vi "FXP Raw to DBL.vi"(7 "FXP Configuration":T1, 8 "error in (no error)":errorcluster, 10 "Bool Data":bool[](array[boolean])) -> (0 "error out":errorcluster, 2 "DBL Value":dbl)   [LabVIEW 2026, in "FPGA Register IO.lvlib"]
uses:
  FPGA Register IO.lvlib
  TypeDefs/FXP Configuration.ctl
  <vilib>/fxp/LVFixedPointRepBitsTypeDef.ctl
  <vilib>/fxp/LVFixedPointRepRangeTypeDef.ctl
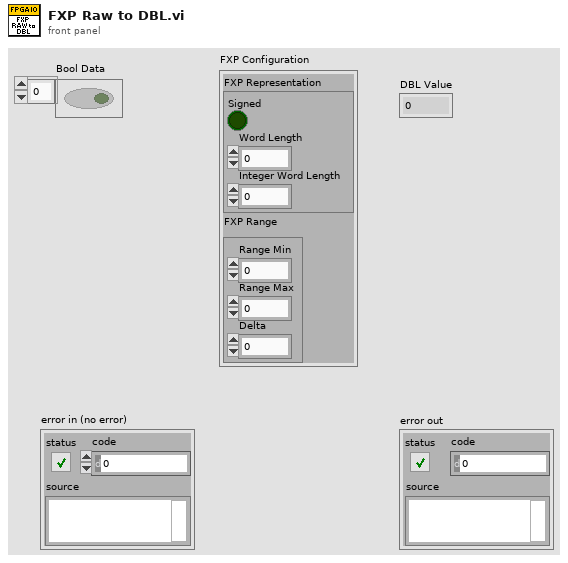
[diagram p1: front panel]
types:
  T1 = typedef "FPGA Register IO.lvlib/FXP Configuration.ctl" = cluster{"FXP Representation":T2, "FXP Range":T3}
  T2 = typedef "LVFixedPointRepBitsTypeDef.ctl" = cluster{"Signed":bool, "Word Length":u32, "Integer Word Length":i32}
  T3 = typedef "LVFixedPointRepRangeTypeDef.ctl" = cluster{"Range Min":dbl, "Range Max":dbl, "Delta":dbl}
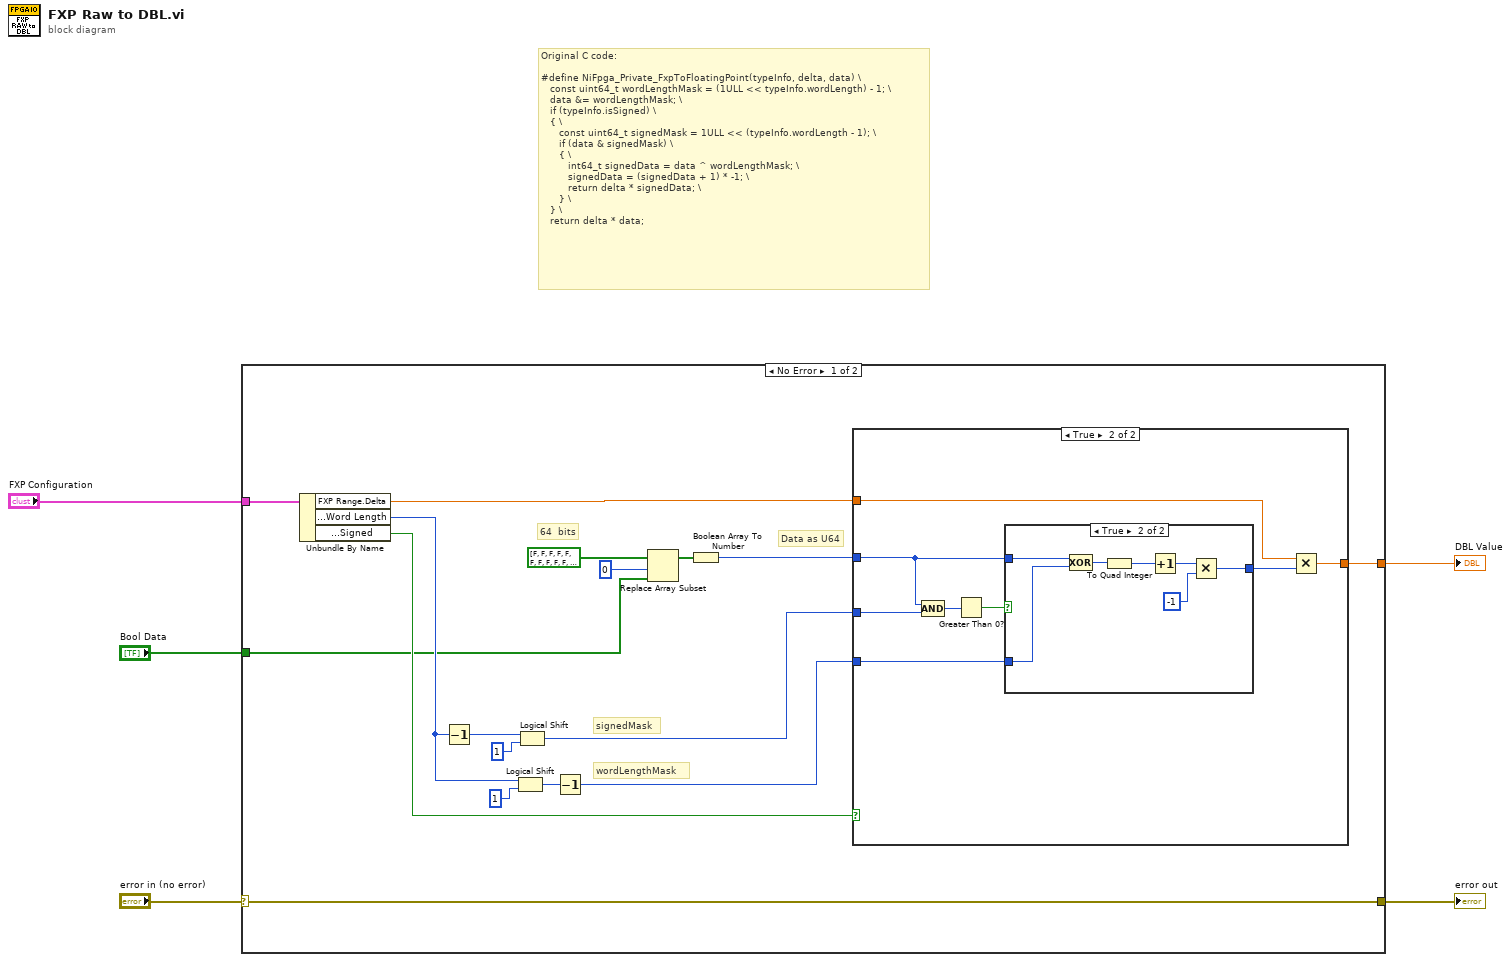
[diagram p0: block diagram]
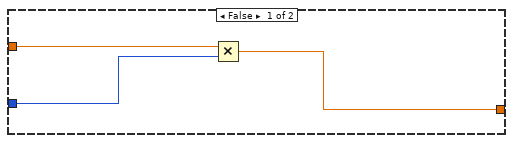
[diagram p2: hidden frame]
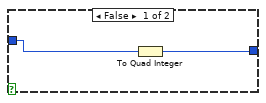
[diagram p3: hidden frame]
diagram:
  # "Original C code: \n\n#define NiFpga_Private_FxpToFloatingPoint(typeInfo, delta, data) \\\n   const uint64_t wordLengthMask = (1ULL << typeInfo.wordLength) - 1; \\\n   data &= wordLengthMask; \\\n   if (typeInfo.isSigned) \\\n   { \\\n      const uint64_t signedMask = 1ULL << (typeInfo.wordLength - 1); \\\n      if (data & signedMask) \\\n      { \\\n         int64_t signedData = data ^ wordLengthMask; \\\n         signedData = (signedData + 1) * -1; \\\n         return delta * signedData; \\\n      } \\\n   } \\\n   return delta * data;"
  n1 = case shown="No Error" "error in (no error)" {
    selector: "error in (no error)" -> [w10 w43]
    tunnel: "Bool Data" -> [w8 _]
    tunnel: [w15 _] -> w3
    tunnel: "FXP Configuration" -> [w14 _]
    tunnel: [w10 w43] -> w2
    frame No Error {
      # "wordLengthMask"
      # "signedMask"
      # "Data as U64"
      # "64  bits"
      n2 = Unbundle By Name(w14) -> ("FXP Range.Delta"=w13:dbl, "FXP Representation.Word Length"=w12:u32, "FXP Representation.Signed"=w11:bool)
      n3 = Decrement(x=w12) -> (x-1=w20:u32)
      n4 = Logical Shift(y=w12, x=u64 1) -> (x << y=w17:u64)
      n5 = Logical Shift(y=w20, x=u64 1) -> (x << y=w19:u64)
      n6 = Decrement(x=w17) -> (x-1=w16:u64)
      n7 = Replace Array Subset(array=bool[] [FALSE, FALSE, FALSE, FALSE, FALSE, FALSE, FALSE, FALSE, FALSE, FALSE, FALSE, FALSE, FALSE, FALSE, FALSE, FALSE, FALSE, FALSE, FALSE, FALSE, FALSE, FALSE, FALSE, FALSE, FALSE, FALSE, FALSE, FALSE, FALSE, FALSE, FALSE, FALSE, FALSE, FALSE, FALSE, FALSE, FALSE, FALSE, FALSE, FALSE, FALSE, FALSE, FALSE, FALSE, FALSE, FALSE, FALSE, FALSE, FALSE, FALSE, FALSE, FALSE, FALSE, FALSE, FALSE, FALSE, FALSE, FALSE, FALSE, FALSE, FALSE, FALSE, FALSE, FALSE], new element=w8, index=0) -> (w6:bool[])
      n8 = Boolean Array To Number(Boolean array=w6) -> (number=w21:u64)
      n9 = case shown="True" w11 {
        tunnel: w21 -> [w24 w30]
        tunnel: w19 -> [_ w33]
        tunnel: w16 -> [_ w29]
        tunnel: w13 -> [w25 w28]
        tunnel: [w23 w27] -> w15
        frame False {
          n10 = Multiply(x=w25, y=w24) -> (x*y=w23:dbl)
        }
        frame True {
          n11 = Compound Arithmetic op=AND(w30, w33) -> (w32:u64)
          n12 = Greater Than 0?(x=w32) -> (x > 0?=w31:bool)
          n13 = case shown="True" w31 {
            tunnel: w30 -> [w34 w42]
            tunnel: w29 -> [_ w41]
            tunnel: [w35 w36] -> w26
            frame False {
              n14 = To Quad Integer(1:w34) -> (0:w35:i64)
            }
            frame True {
              n15 = Compound Arithmetic op=XOR(w42, w41) -> (w40:u64)
              n16 = To Quad Integer(1:w40) -> (0:w39:i64)
              n17 = Increment(x=w39) -> (x+1=w38:i64)
              n18 = Multiply(x=w38, y=i64 -1) -> (x*y=w36:i64)
            }
          }
          n19 = Multiply(x=w28, y=w26) -> (x*y=w27:dbl)
        }
      }
    }
    frame Error {
    }
  }
  "DBL Value" <- w3
  "error out" <- w2
